vi "SDSU_SetDacsHw.vi"(0 "fd":i32, 1 "board":string, 2 "dac number":string, 3 "type":string, 4 "dac value":string, 5 "error IO":errorcluster, 7 "volts value":string, 8 "dac array":string[][](array[string]), 9 "index":i32, 11 "current index":u8) -> (14 "fd out":i32, 15 "dac array out":string[][](array[string]), 17 "response":string, 19 "error IO 2":errorcluster)   [LabVIEW 2016]
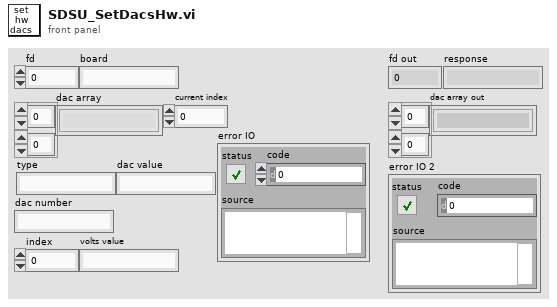
[diagram p1: front panel]
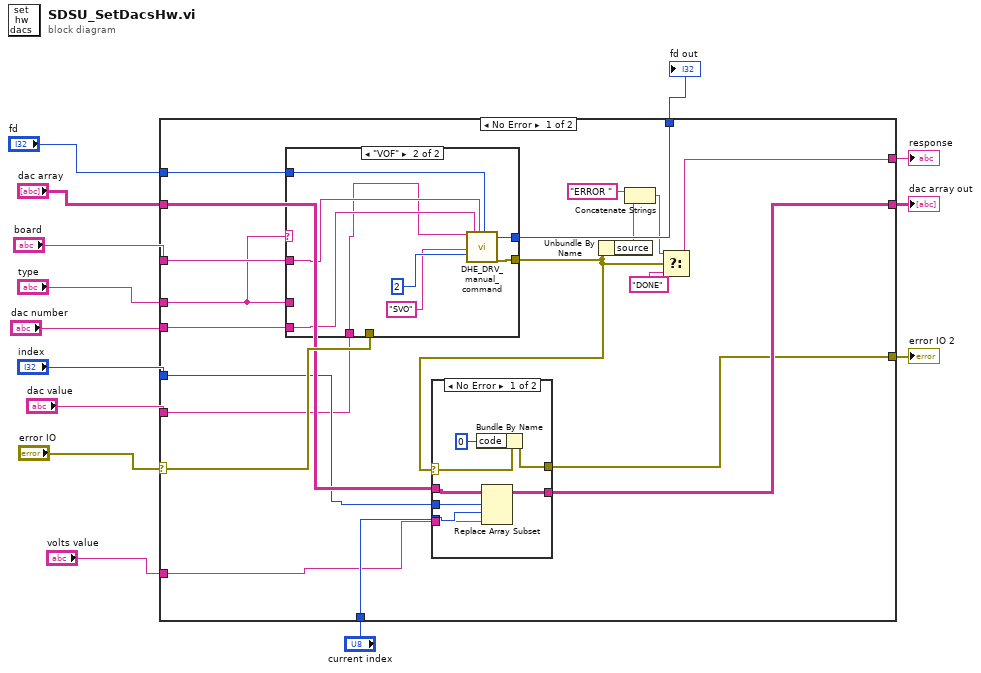
[diagram p0: block diagram]
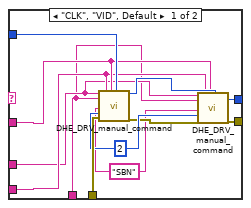
[diagram p2: hidden frame]
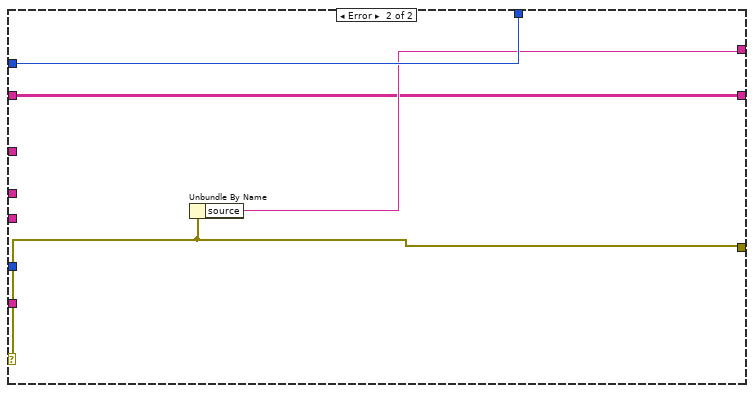
[diagram p4: hidden frame]
diagram:
  n1 = case shown="No Error" "error IO" {
    selector: "error IO" -> [w30 w66]
    tunnel: "fd" -> [w33 w67]
    tunnel: [w23 w67] -> w5
    tunnel: [w24 w66] -> w2
    tunnel: [w31 w65] -> w1
    tunnel: "type" -> [w15 _]
    tunnel: "board" -> [w21 _]
    tunnel: "dac number" -> [w20 _]
    tunnel: "dac value" -> [w16 _]
    tunnel: "dac array" -> [w29 w64]
    tunnel: [w26 w64] -> w3
    tunnel: "index" -> [w28 _]
    tunnel: "current index" -> [w27 _]
    tunnel: "volts value" -> [w25 _]
    frame No Error {
      n2 = case shown="\"VOF\"" w15 {
        tunnel: w33 -> [w45 w47]
        tunnel: w30 -> [w44 _]
        tunnel: [w40 w52] -> w23
        tunnel: [w39 w51] -> w22
        tunnel: w21 -> [w37 w49]
        tunnel: w20 -> [w36 w48]
        tunnel: w15 -> [w35 _]
        tunnel: w16 -> [w34 w46]
        frame "CLK", "VID", Default {
          w43 = i16 2 ("short board_dest")
          w38 = "SBN" ("command")
          n3 = call "DHE_DRV_manual_command.vi"("arg3"=w35, "arg4"=w34, "command"=w38, "short board_dest"=w43, "error in (no error)"=w44, "arg2"=w36, "arg1"=w37, "fd"=w45) -> ("fd"=w41:i32, "error out"=w42:errorcluster)  [unwired: 1 in, 9 out]
          n4 = call "DHE_DRV_manual_command.vi"("arg3"=w35, "arg4"=w34, "command"=w38, "short board_dest"=w43, "error in (no error)"=w42, "arg2"=w36, "arg1"=w37, "fd"=w41) -> ("fd"=w40:i32, "error out"=w39:errorcluster)  [unwired: 1 in, 9 out]
        }
        frame "VOF" {
          n5 = call "DHE_DRV_manual_command.vi"("arg3"=w46, "command"="SVO", "short board_dest"=i16 2, "arg2"=w48, "arg1"=w49, "fd"=w47) -> ("fd"=w52:i32, "error out"=w51:errorcluster)  [unwired: 3 in, 9 out]
        }
      }
      n6 = case shown="No Error" w22 {
        selector: w22 -> [w55 w62]
        tunnel: w29 -> [w61 w63]
        tunnel: w28 -> [w60 _]
        tunnel: w27 -> [w59 _]
        tunnel: [w58 w63] -> w26
        tunnel: w25 -> [w57 _]
        tunnel: [w54 w62] -> w24
        frame No Error {
          n7 = Bundle By Name(cluster=w55, "code"=0) -> (w54:errorcluster)
          n8 = Replace Array Subset(array=w61, new element=w57, index (row)=w60, index (col)=w59) -> (w58:string[][])
        }
        frame Error {
        }
      }
      n9 = Unbundle By Name(w22) -> ("source"=w17:string)
      n10 = Concatenate Strings("ERROR " ("string"), w17) -> (w18:string)
      n11 = Select(t=w18, s=w22, f="DONE") -> (s? t:f=w31:string)
    }
    frame Error {
      n12 = Unbundle By Name(w66) -> ("source"=w65:string)
    }
  }
  "fd out" <- w5
  "dac array out" <- w3
  "error IO 2" <- w2
  "response" <- w1
